vi "turn_off_Magnet_and_set_persitent.vi"   [LabVIEW 2019]
uses:
  Instrument_Setup.vi
  Monitors/Utility/Monitor Communication/sub-vis/16T_Open_Queue.vi
  Global/Global Variables/Data_Display_global.vi
  Monitors/Utility/Monitor Communication/sub-vis/16T_Split_Cluster.vi
  Monitors/Utility/Monitor Communication/sub-vis/16T_Queue_Commands.vi
  Monitors/Utility/Monitor Communication/sub-vis/20T_Open_Queue.vi
  Monitors/Utility/Monitor Communication/sub-vis/20T_Split_Cluster.vi
  Monitors/Utility/Monitor Communication/sub-vis/20T_Queue_Commands.vi
types:
  T1 = typedef "16T-Cluster.ctl" = cluster{"Clamp":bool, "Switch Heater":bool, "Go to Zero":bool, "Go to set":bool, "Go to Hold":bool, "Clamped":bool, "Quenched":bool, "Rate limit":bool, "Persistent":bool, "Hold":bool, "Set":bool, "Zero":bool, "Magnet (T)":dbl, "Leads (T)":dbl, "Magnet T (K)":dbl, "Switch":bool, "Setpoint (T)":dbl, "Rate (T/min)":dbl, "Select":bool, "Sweeping":bool}
  T2 = typedef "16T_Control.ctl" = cluster{"Clamp":bool, "Switch Heater":bool, "Go to Zero":bool, "Go to Set":bool, "Go to Hold":bool, "Setpoint (T)":dbl, "Rate (T/min)":dbl, "Set Rate":bool}
  T3 = typedef "15T-Cluster.ctl" = cluster{"Magnet (T)":dbl, "Leads (T)":dbl, "Setpoint (T)":dbl, "Rate (T/min)":dbl, "Set":bool, "Zero":bool, "Hold":bool, "Go to zero":bool, "Go to Hold":bool, "Go to Set":bool, "Clamp":bool, "Switch Heater":bool, "Rate limit":bool, "Switch":bool, "Clamped":bool, "Persistent":bool, "Quenched":bool, "Sweeping":bool, "Select":bool}
  T4 = typedef "15T-Control.ctl" = cluster{"Setpoint (T)":dbl, "Rate (T/min)":dbl, "Go to zero":bool, "Go to Hold":bool, "Go to Set":bool, "Clamp":bool, "Switch Heater":bool}
  T5 = typedef "20T_Cluster.ctl" = cluster{"Clamp":bool, "Switch Heater":bool, "Go to Zero":bool, "Go to set":bool, "Go to Hold":bool, "Clamped":bool, "Hold":bool, "Set":bool, "Zero":bool, "Magnet (T)":dbl, "Leads (T)":dbl, "Magnet T (K)":dbl, "Switch":bool, "Target Field (T)":dbl, "Field Setpoint (T)":dbl, "Rate Setpoint (T/min)":dbl, "Set Rate":bool, "Rate\n(T/min) ":dbl, "lambda NV (%)":dbl, "lambda p (mbar)":dbl, "lambda-Control":bool, "Activate lambda control":bool, "lambda NV  SP":dbl, "Set lambda NV":bool, "PSU Status":string, "PSU\nVoltage":dbl}
  T6 = typedef "20T_Control.ctl" = cluster{"Clamp":bool, "Switch Heater":bool, "Go to Zero":bool, "Go to Set":bool, "Go to Hold":bool, "Field Setpoint (T)":dbl, "Rate Setpoint (T/min)":dbl, "Set Rate":bool, "Activate lambda control":bool, "Set lambda NV":bool, "lambda NV  SP":dbl}
  T7 = typedef "5T-Cluster.ctl" = cluster{"Go to set":bool, "Go to Zero":bool, "Clamp":bool, "Go to Hold":bool, "Clamped ":bool, "Quenched 2":bool, "Rate limit 2":bool, "Magnet (T)":dbl, "Leads (T)":dbl, "Rate (T/min)":dbl, "Sweeping":bool, "Setpoint":dbl, "Set":bool, "Zero":bool, "Hold":bool, "Clamp":bool}
  T8 = typedef "5T_Control.ctl" = cluster{"Rate (T/min)":dbl, "Setpoint":dbl, "Go to set":bool, "Go to Zero":bool, "Clamp":bool, "Go to Hold":bool, "Set Rate":bool}
  T9 = typedef "P9_P14_Magnet-cluster.ctl" = cluster{"Magnet (Oe)":dbl, "Setpoint (Oe)":dbl, "Rate (Oe/min)":dbl, "Set Field":bool, "Go to zero":bool, "Set Persitant/non-pers":bool, "Approach":i32, "Magnet Status":i32, "Sweeping":bool, "Quenched":bool, "Persitant Mode ":bool, "Stable":bool, "Steps":dbl, "Paused Menu":dbl, "B Step Start Field":dbl}
  T10 = typedef "P9P14_Magnet_Control.ctl" = cluster{"Setpoint (Oe)":dbl, "Rate (Oe/min)":dbl, "Set Field":bool, "Go to zero":bool, "Set Persitant/non-pers":bool, "Approach":i32, "Steps":dbl, "Paused Menu":dbl, "B Step start Field":dbl}
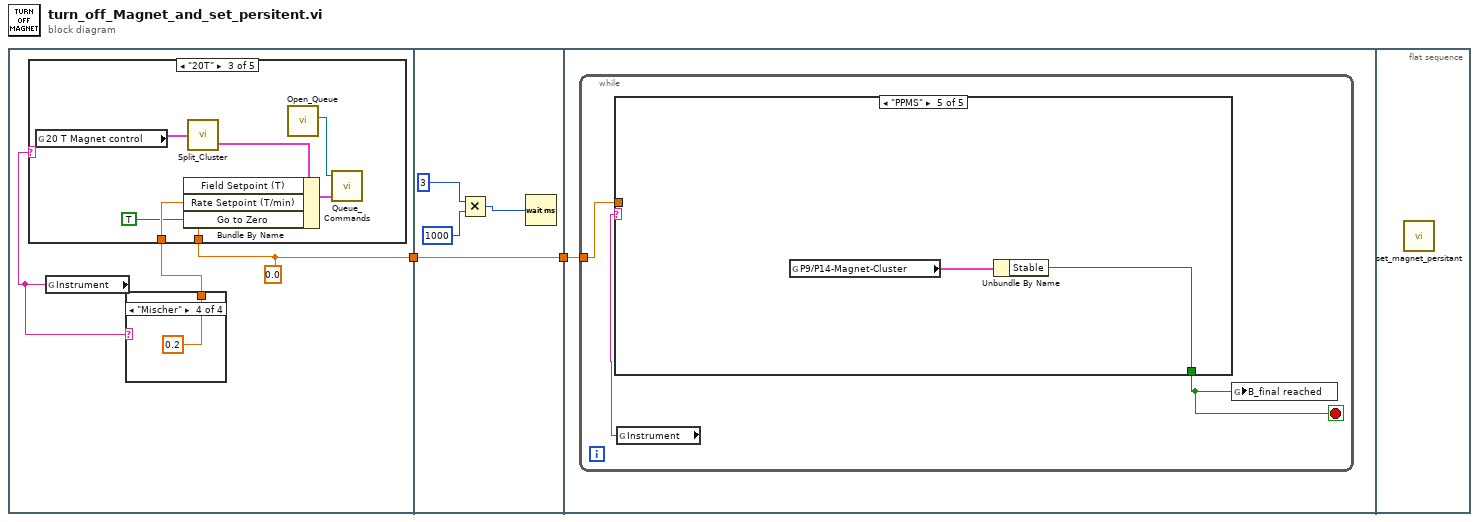
[diagram p0: block diagram]
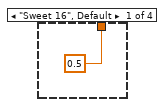
[diagram p2: hidden frame]
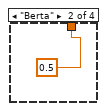
[diagram p3: hidden frame]
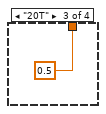
[diagram p4: hidden frame]
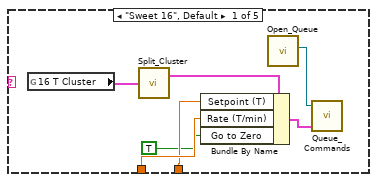
[diagram p5: hidden frame]
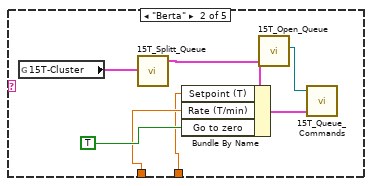
[diagram p6: hidden frame]
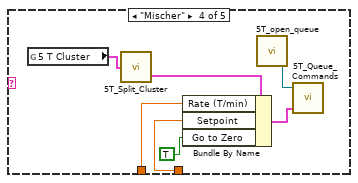
[diagram p7: hidden frame]
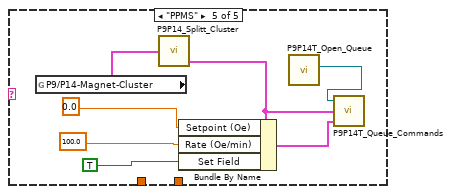
[diagram p8: hidden frame]
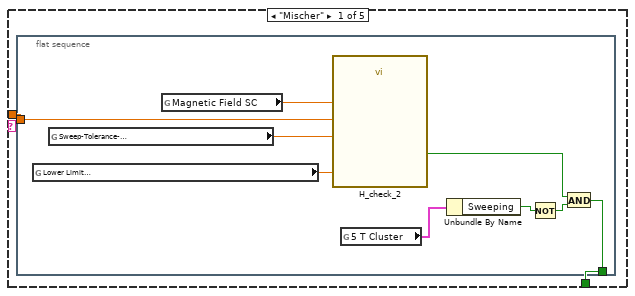
[diagram p9: hidden frame]
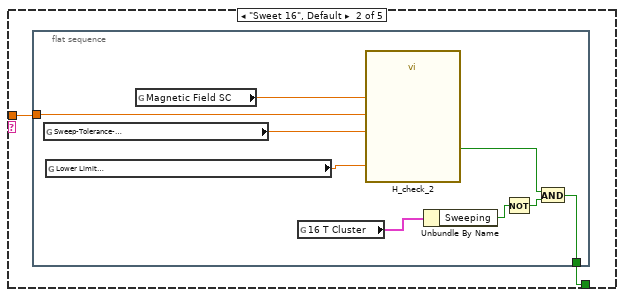
[diagram p10: hidden frame]
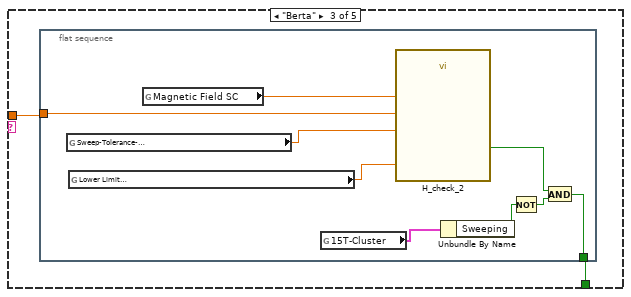
[diagram p11: hidden frame]
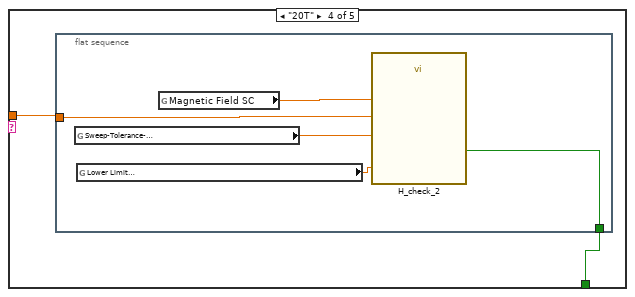
[diagram p12: hidden frame]
diagram:
  n1 = flat-sequence {
    tunnel: [w3] -> w2
    tunnel: w2 -> [w48]
    tunnel: [w48] -> w1
    tunnel: w1 -> [w49]
    frame #0 {
      w3 = 0.0
      n2 = global read "Instrument_Setup.vi" "Instrument"() -> (w4:string)
      n3 = case shown="\"Mischer\"" w4 {
        tunnel: [0.5 0.5 0.5 0.2] -> w5
        frame "Sweet 16", Default {
        }
        frame "Berta" {
        }
        frame "20T" {
        }
        frame "Mischer" {
        }
      }
      n4 = case shown="\"20T\"" w4 {
        tunnel: w5 -> [w14 w18 w26 w32 _]
        tunnel: w3 -> [w13 w17 w25 w31 _]
        frame "Sweet 16", Default {
          n5 = global read "Data_Display_global.vi" "16 T Cluster"() -> (w15:T1)
          n6 = call-poly "Split_Cluster.vi"("16 T Magnet control"=w15) -> ("16 T Magnet control"=w12:T2)  [unwired: 1 out]
          n7 = Bundle By Name(cluster=w12, "Setpoint (T)"=w13, "Rate (T/min)"=w14, "Go to Zero"=TRUE) -> (w11:T2)
          n8 = call-poly "Open_Queue.vi"() -> ("queue out"=w16:refnum<queue>)  [unwired: 10 in, 1 out]
          n9 = call-poly "Queue_Commands.vi"("16 T Magnet control"=w11, "16T Queue"=w16) -> ()  [unwired: 1 in, 1 out]
        }
        frame "Berta" {
          n10 = global read "Data_Display_global.vi" "15T-Cluster"() -> (w22:T3)
          n11 = call "15T_Splitt_Queue.vi"("15T-Cluster"=w22) -> ("15T-Control"=w21:T4)  [unwired: 1 in, 1 out]
          n12 = Bundle By Name(cluster=w21, "Setpoint (T)"=w17, "Rate (T/min)"=w18, "Go to zero"=TRUE) -> (w19:T4)
          n13 = call "15T_Open_Queue.vi"() -> ("queue out"=w23:refnum<queue>)  [unwired: 10 in, 1 out]
          n14 = call "15T_Queue_Commands.vi"("15T-Control"=w19, "15T Queue"=w23) -> ()  [unwired: 1 in, 1 out]
        }
        frame "20T" {
          n15 = global read "Data_Display_global.vi" "20 T Magnet control"() -> (w29:T5)
          n16 = call-poly "Split_Cluster.vi"("20 T Cluster"=w29) -> ("20 T Control"=w27:T6)  [unwired: 1 out]
          n17 = Bundle By Name(cluster=w27, "Field Setpoint (T)"=w25, "Rate Setpoint (T/min)"=w26, "Go to Zero"=TRUE) -> (w28:T6)
          n18 = call-poly "Open_Queue.vi"() -> ("queue out"=w30:refnum<queue>)  [unwired: 10 in, 1 out]
          n19 = call-poly "Queue_Commands.vi"("20T Control (in)"=w28, "20T Queue"=w30) -> ()  [unwired: 1 in, 1 out]
        }
        frame "Mischer" {
          n20 = global read "Data_Display_global.vi" "5 T Cluster"() -> (w37:T7)
          n21 = call "5T_Split_Cluster.vi"("5 T Cluster"=w37) -> ("5T Control"=w36:T8)  [unwired: 1 out]
          n22 = Bundle By Name(cluster=w36, "Rate (T/min)"=w32, "Setpoint"=w31, "Go to Zero"=TRUE) -> (w35:T8)
          n23 = call "5T_open_queue.vi"() -> ("queue out"=w34:refnum<queue>)  [unwired: 10 in, 1 out]
          n24 = call "5T_Queue_Commands.vi"("5T Control"=w35, "5T Queue"=w34) -> ()  [unwired: 1 in, 1 out]
        }
        frame "PPMS" {
          n25 = global read "Data_Display_global.vi" "P9/P14-Magnet-Cluster"() -> (w44:T9)
          n26 = call "P9P14_Splitt_Cluster.vi"("P9/P14-Magnet-Cluster"=w44) -> ("P9/P14-Magnet-Control"=w43:T10)  [unwired: 1 in, 1 out]
          n27 = Bundle By Name(cluster=w43, "Setpoint (Oe)"=0.0, "Rate (Oe/min)"=100.0, "Set Field"=TRUE) -> (w41:T10)
          n28 = call "P9P14T_Open_Queue.vi"() -> ("queue out"=w40:refnum<queue>)  [unwired: 10 in, 1 out]
          n29 = call "P9P14T_Queue_Commands.vi"("P9/P14-Magnet-Control"=w41, "P9/P14-Magnet-Control old status"=w43, "16T Queue"=w40) -> ()  [unwired: 1 out]
        }
      }
    }
    frame #1 {
      n30 = Multiply(x=3, y=1000) -> (x*y=w47:i32)
      n31 = Wait (ms)(milliseconds to wait=w47) -> ()  [unwired: 1 out]
    }
    frame #2 {
      n32 = while {
        tunnel: w49 -> [w52]
        stop <- w51 stop-if-true
        n33 = global read "Instrument_Setup.vi" "Instrument"() -> (w50:string)
        n34 = case shown="\"PPMS\"" w50 {
          tunnel: [w53 w65 w76 w86 w93] -> w51
          tunnel: w52 -> [w54 w64 w75 w87 _]
          frame "Mischer" {
            n35 = flat-sequence {
              tunnel: [w58] -> w53
              tunnel: w54 -> [w61]
              frame #0 {
                n36 = global read "Instrument_Setup.vi" "Lower Limit\nSweep-Tolerance-\nMagnetic-Field (T)"() -> (w55:dbl)
                n37 = global read "Instrument_Setup.vi" "Sweep-Tolerance-\nMagnetic-Field (%)"() -> (w63:dbl)
                n38 = global read "Data_Display_global.vi" "Magnetic Field SC"() -> (w62:dbl)
                n39 = call "H_check_2.vi"("Lower Limit\nSweep\nTolerance (T)"=w55, "Sweep\nTolerance %"=w63, "H_in"=w62, "H_target (K)"=w61) -> ("= H target"=w59:bool)  [unwired: 7 in]
                n40 = global read "Data_Display_global.vi" "5 T Cluster"() -> (w60:T7)
                n41 = Unbundle By Name(w60) -> ("Sweeping"=w56:bool)
                n42 = Not(x=w56) -> (.not. x?=w57:bool)
                n43 = And(x=w59, y=w57) -> (x .and. y?=w58:bool)
              }
            }
          }
          frame "Sweet 16", Default {
            n44 = flat-sequence {
              tunnel: [w70] -> w65
              tunnel: w64 -> [w73]
              frame #0 {
                n45 = global read "Instrument_Setup.vi" "Sweep-Tolerance-\nMagnetic-Field (%)"() -> (w67:dbl)
                n46 = global read "Instrument_Setup.vi" "Lower Limit\nSweep-Tolerance-\nMagnetic-Field (T)"() -> (w66:dbl)
                n47 = global read "Data_Display_global.vi" "Magnetic Field SC"() -> (w74:dbl)
                n48 = global read "Data_Display_global.vi" "16 T Cluster"() -> (w72:T1)
                n49 = call "H_check_2.vi"("Lower Limit\nSweep\nTolerance (T)"=w66, "Sweep\nTolerance %"=w67, "H_in"=w74, "H_target (K)"=w73) -> ("= H target"=w71:bool)  [unwired: 7 in]
                n50 = Unbundle By Name(w72) -> ("Sweeping"=w68:bool)
                n51 = Not(x=w68) -> (.not. x?=w69:bool)
                n52 = And(x=w71, y=w69) -> (x .and. y?=w70:bool)
              }
            }
          }
          frame "Berta" {
            n53 = flat-sequence {
              tunnel: [w81] -> w76
              tunnel: w75 -> [w84]
              frame #0 {
                n54 = global read "Instrument_Setup.vi" "Sweep-Tolerance-\nMagnetic-Field (%)"() -> (w78:dbl)
                n55 = global read "Instrument_Setup.vi" "Lower Limit\nSweep-Tolerance-\nMagnetic-Field (T)"() -> (w77:dbl)
                n56 = global read "Data_Display_global.vi" "Magnetic Field SC"() -> (w85:dbl)
                n57 = global read "Data_Display_global.vi" "15T-Cluster"() -> (w83:T3)
                n58 = call "H_check_2.vi"("Lower Limit\nSweep\nTolerance (T)"=w77, "Sweep\nTolerance %"=w78, "H_in"=w85, "H_target (K)"=w84) -> ("= H target"=w82:bool)  [unwired: 7 in]
                n59 = Unbundle By Name(w83) -> ("Sweeping"=w79:bool)
                n60 = Not(x=w79) -> (.not. x?=w80:bool)
                n61 = And(x=w82, y=w80) -> (x .and. y?=w81:bool)
              }
            }
          }
          frame "20T" {
            n62 = flat-sequence {
              tunnel: [w90] -> w86
              tunnel: w87 -> [w91]
              frame #0 {
                n63 = global read "Instrument_Setup.vi" "Sweep-Tolerance-\nMagnetic-Field (%)"() -> (w89:dbl)
                n64 = global read "Instrument_Setup.vi" "Lower Limit\nSweep-Tolerance-\nMagnetic-Field (T)"() -> (w88:dbl)
                n65 = global read "Data_Display_global.vi" "Magnetic Field SC"() -> (w92:dbl)
                n66 = call "H_check_2.vi"("Lower Limit\nSweep\nTolerance (T)"=w88, "Sweep\nTolerance %"=w89, "H_in"=w92, "H_target (K)"=w91) -> ("= H target"=w90:bool)  [unwired: 7 in]
              }
            }
          }
          frame "PPMS" {
            n67 = global read "Data_Display_global.vi" "P9/P14-Magnet-Cluster"() -> (w94:T9)
            n68 = Unbundle By Name(w94) -> ("Stable"=w93:bool)
          }
        }
        n69 = global write "Data_Display_global.vi" "B_final reached"(w51) -> ()
      }
    }
    frame #3 {
      n70 = call "set_magnet_persitant.vi"() -> ()  [unwired: 4 in]
    }
  }
